vi "FSK - Sender.vi"(8 "error in (no error)":errorcluster, 11 "Queues":T1) -> (0 "error out":errorcluster)   [LabVIEW 2013]
uses:
  <vilib>/sound2/lvsound2.llb/Sound Output Task ID.ctl
  <vilib>/sound2/lvsound2.llb/Sound Data Format.ctl
  STYPS/HDR - Queues.ctl
  <vilib>/sound2/lvsound2.llb/Sampling Mode.ctl
  <vilib>/sound2/lvsound2.llb/Sound Output Write (DBL Single).vi
panel:
  out "string":string
  in  "Play Button":bool
  out "Array":u8[](array[numeric])
  in  "data length (B)":i32=100
  in  "PROPERTIES":T4={"device ID"=0, "number of samples/ch"=2500, "task ID"=0, "sound format"={"sample rate (S/s)"=44100.0, "number of channels"=1, "bits per sample"=16}, "DATA"=[]} {"task ID" format="%.0x"}
  out "i":i32
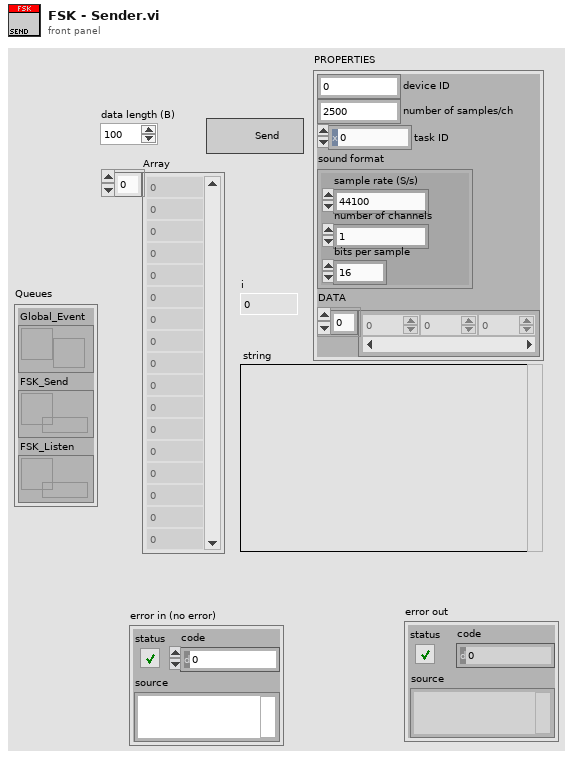
[diagram p1: front panel]
types:
  T1 = typedef "HDR - Queues.ctl" = cluster{"Global_Event":refnum<user-event>, "FSK_Send":refnum<queue>, "FSK_Listen":refnum<queue>}
  T2 = typedef "Sound Output Task ID.ctl" = u32
  T3 = typedef "Sound Data Format.ctl" = cluster{"sample rate (S/s)":dbl, "number of channels":i32, "bits per sample":i32}
  T4 = cluster{"device ID":u32, "number of samples/ch":i32, "task ID":T2, "sound format":T3, "DATA":dbl[]}
  T5 = typedef "Sampling Mode.ctl" = i32
  T6 = typedef "FSK_OBJ - PROP.ctl" = cluster{"rate (bit/s)":dbl, "bp (Bit Period)":dbl, "f1%":dbl, "f2%":dbl, "f1 (1 Freq)":dbl, "f2 (0 Freq)":dbl, "t (Time arry)":dbl[], "y1 (f1 cos arry)":dbl[], "y2 (f2 cos arry)":dbl[], "data length (B)":i32, "data size":i32, "sample size":dbl}
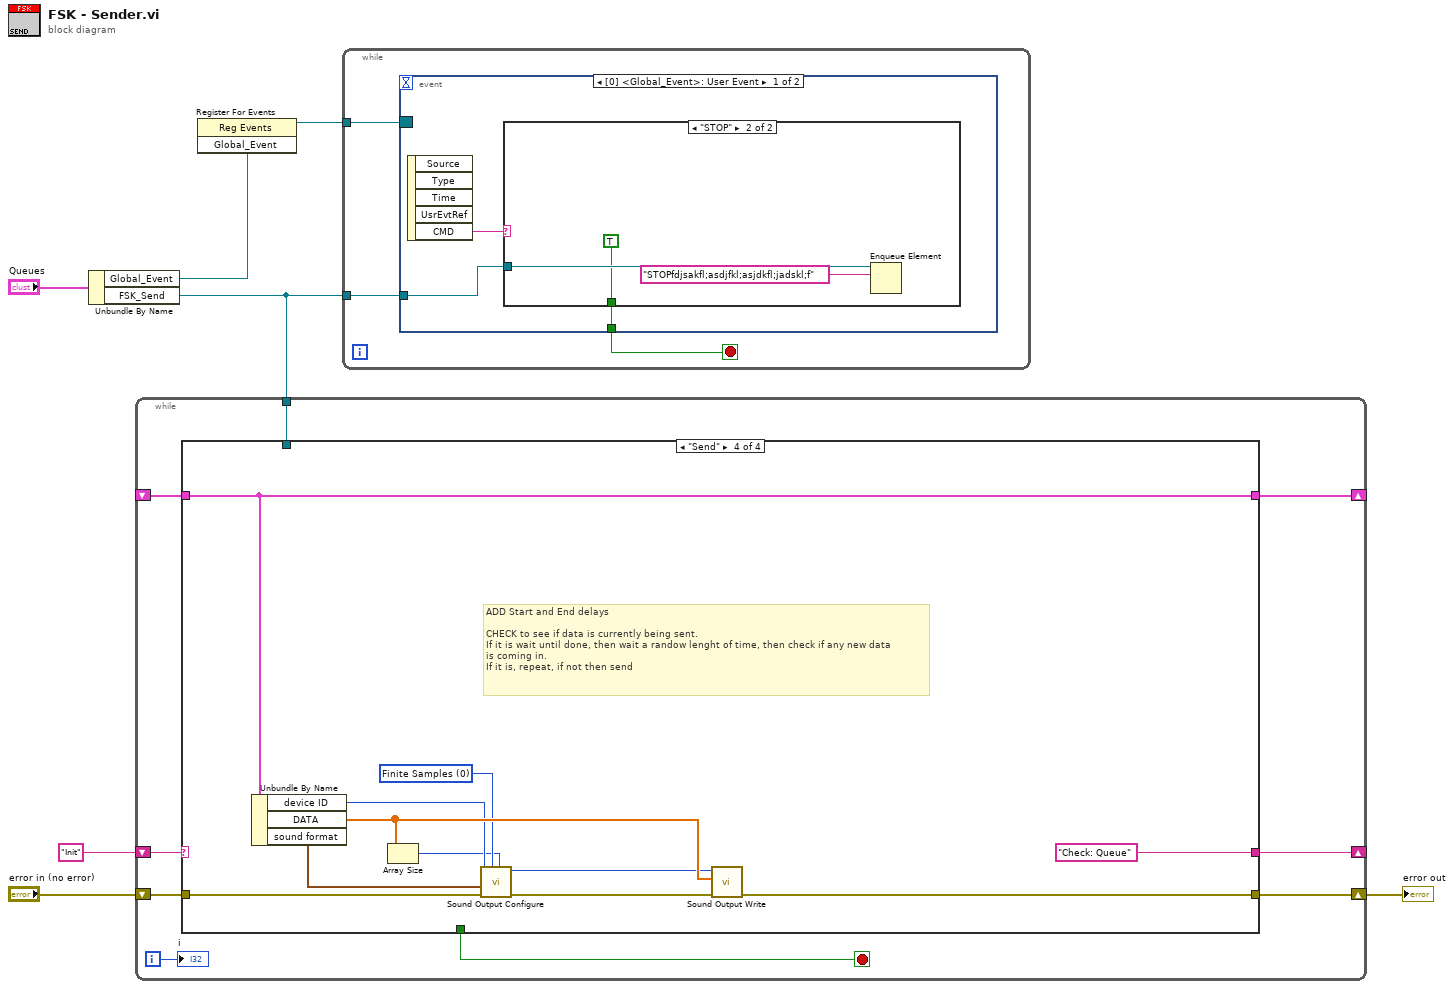
[diagram p0: block diagram]
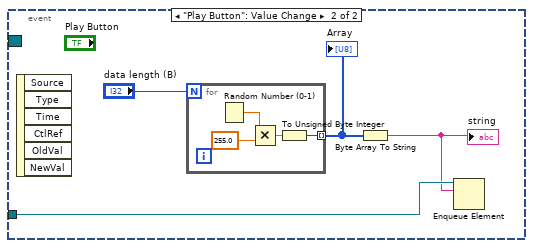
[diagram p3: hidden frame]
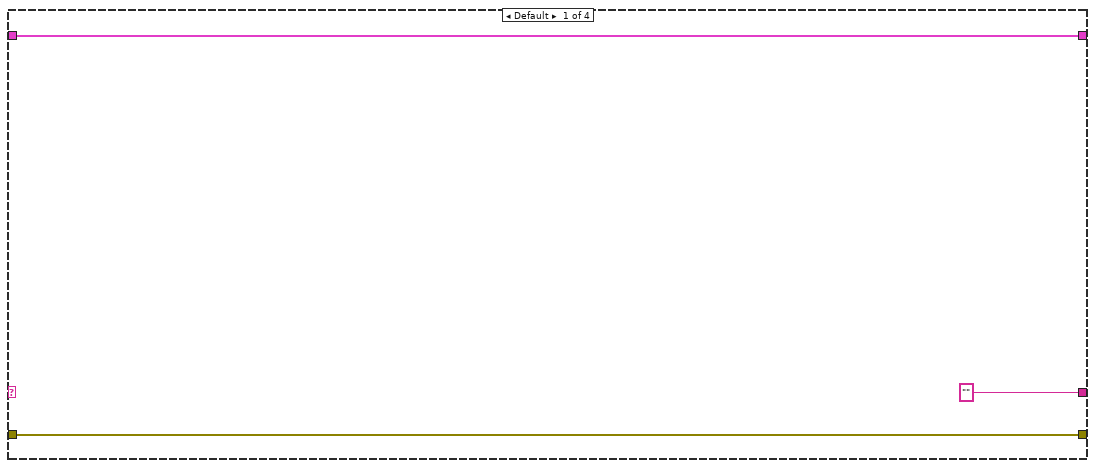
[diagram p4: hidden frame]
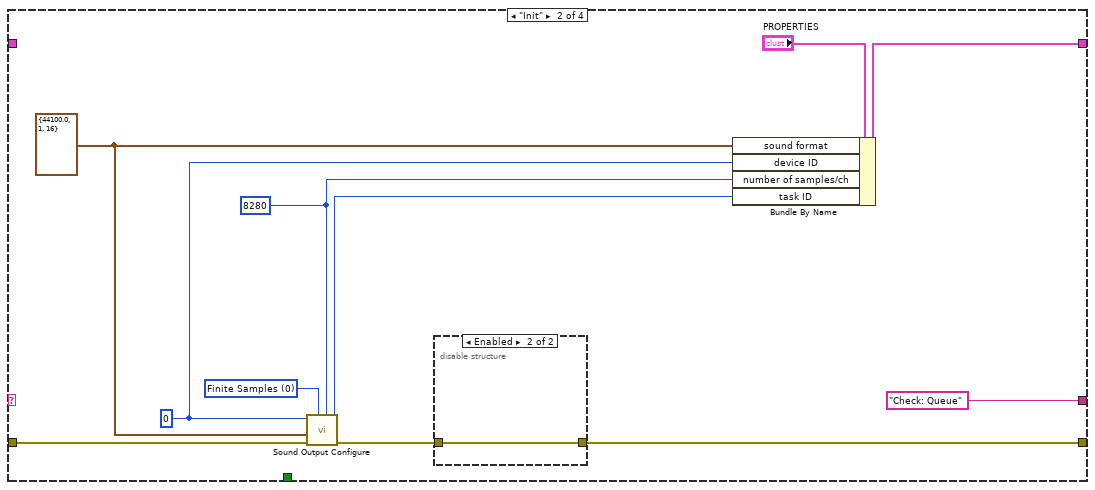
[diagram p5: hidden frame]
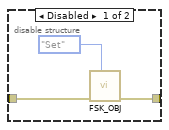
[diagram p6: hidden frame]
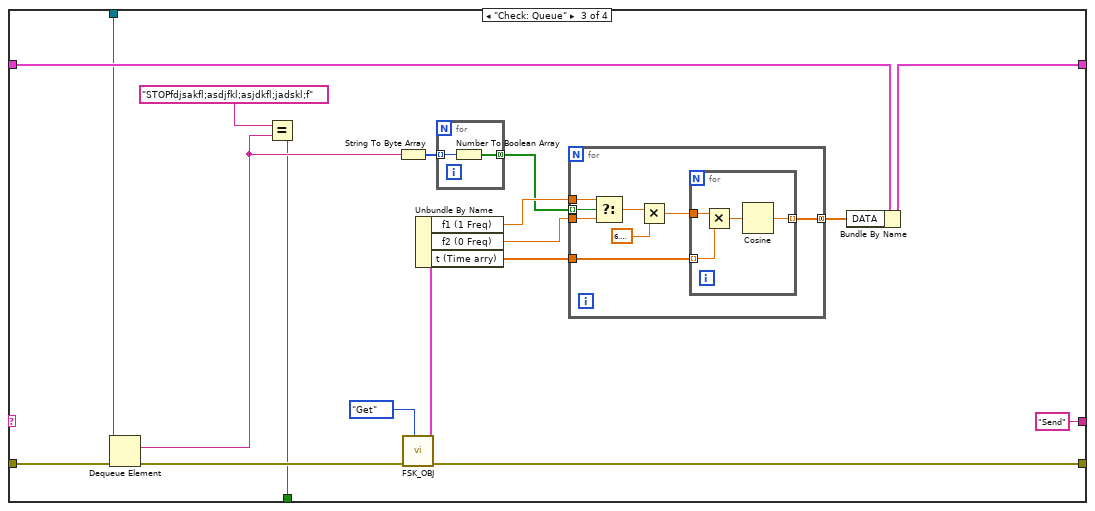
[diagram p7: hidden frame]
diagram:
  n1 = Unbundle By Name("Queues") -> ("Global_Event"=w3:refnum<user-event>, "FSK_Send"=w5:refnum<queue>)
  n2 = while {
    shift-right: [w13] -> _
    shift-left: "Init" -> [w14]
    shift-right: [w12] -> w1
    shift-left: "error in (no error)" -> [w16]
    shift-right: [w11] -> _
    shift-left: _ -> [w10]
    tunnel: w5 -> [w9]
    i -> [w15]
    stop <- w8 stop-if-true
    n3 = case shown="\"Send\"" w14 {
      tunnel: w16 -> [w19 w29 w42 w73]
      tunnel: ["" "Check: Queue" "Send" "Check: Queue"] -> w13
      tunnel: [w19 w20 w50 w76] -> w12
      tunnel: [w18 w26 w40 w75] -> w11
      tunnel: w10 -> [w18 _ w52 w75]
      tunnel: w9 -> [_ _ w38 _]
      tunnel: [_ _ w35 _] -> w8
      frame Default {
      }
      frame "Init" {
        w23 = u32 0 ("device ID")
        w24 = T3 {"sample rate (S/s)"=44100.0, "number of channels"=1, "bits per sample"=16} ("sound format")
        w25 = 8280 ("number of samples/ch")
        w30 = T5 0 items=["Finite Samples", "Continuous Samples"] ("sample mode")
        n4 = call <vilib>:"Sound Output Configure.vi"("number of samples/ch"=w25, "sample mode"=w30, "error in (no error)"=w29, "sound format"=w24, "device ID"=w23) -> ("error out"=w21:errorcluster, "task ID"=w22:T2)  [unwired: 5 in]
        n5 = disable-structure shown="Enabled" {
          disable-tunnel: w21 -> [w33 w34]
          disable-tunnel: [w32 w34] -> w20
          frame Disabled {
            n6 = call "FSK_OBJ.vi"("Mode"=enum16{"Get", "Set"}."Set", "error in"=w33) -> ("error out"=w32:errorcluster)  [unwired: 8 in, 1 out]
          }
          frame Enabled {
          }
        }
        n7 = Bundle By Name(cluster="PROPERTIES", "sound format"=w24, "device ID"=w23, "number of samples/ch"=w25, "task ID"=w22) -> (w26:T4)
      }
      frame "Check: Queue" {
        n8 = Dequeue Element(queue=w38, error in (no error)=w42) -> (element=w37:string, error out=w41:errorcluster)  [unwired: 1 in, 2 out]
        n9 = Equal?(x="STOPfdjsakfl;asdjfkl;asjdkfl;jadskl;f" ("element"), y=w37) -> (x = y?=w35:bool)
        n10 = String To Byte Array(string=w37) -> (unsigned byte array=w44:u8[])
        n11 = call "FSK_OBJ.vi"("Mode"=enum16{"Get", "Set"}."Get", "error in"=w41) -> ("error out"=w50:errorcluster, "PROPERTIES OUT"=w48:T6)  [unwired: 8 in]
        n12 = Unbundle By Name(w48) -> ("f1 (1 Freq)"=w46:dbl, "f2 (0 Freq)"=w45:dbl, "t (Time arry)"=w47:dbl[])
        n13 = for {
          tunnel: w44 -> [w54] mode=indexing
          tunnel: [w53] -> w43 mode=concatenating
          n14 = Number To Boolean Array(number=w54) -> (Boolean array=w53:bool[])
        }
        n15 = for {
          tunnel: w43 -> [w62] mode=indexing
          tunnel: w47 -> [w56]
          tunnel: w46 -> [w61]
          tunnel: w45 -> [w60]
          tunnel: [w55] -> w39 mode=concatenating
          n16 = Select(t=w61, s=w62, f=w60) -> (s? t:f=w59:dbl)
          n17 = Multiply(x=w59, y=6.283185307179586) -> (x*y=w57:dbl)
          n18 = for {
            tunnel: w57 -> [w66]
            tunnel: w56 -> [w65] mode=indexing
            tunnel: [w63] -> w55 mode=indexing
            n19 = Multiply(x=w66, y=w65) -> (x*y=w64:dbl)
            n20 = Cosine(x=w64) -> (cos(x)=w63:dbl)
          }
        }
        n21 = Bundle By Name(cluster=w52, "DATA"=w39) -> (w40:T4)
      }
      frame "Send" {
        w69 = T5 0 items=["Finite Samples", "Continuous Samples"] ("sample mode")
        # "ADD Start and End delays\n\nCHECK to see if data is currently being sent.\nIf it is wait until done, then wait a randow lenght of time, then check if any new data\nis coming in.\nIf it is, repeat, if not then send"
        n22 = Unbundle By Name(w75) -> ("device ID"=w70:u32, "DATA"=w74:dbl[], "sound format"=w67:T3)
        n23 = Array Size(array=w74) -> (size(s)=w68:i32)
        n24 = call <vilib>:"Sound Output Configure.vi"("number of samples/ch"=w68, "sample mode"=w69, "error in (no error)"=w73, "sound format"=w67, "device ID"=w70) -> ("error out"=w72:errorcluster, "task ID"=w71:T2)  [unwired: 5 in]
        n25 = call-poly <vilib>:"Sound Output Write.vi"("error in (no error)"=w72, "data"=w74, "task ID"=w71) -> ("error out"=w76:errorcluster)  [unwired: 7 in, 1 out]
      }
    }
    "i" <- w15
  }
  "error out" <- w1
  n26 = register-events(w3) -> (reference out=w2:refnum<event-registration>)  [unwired: 2 in, 1 out]
  n27 = while {
    tunnel: w5 -> [w80]
    tunnel: w2 -> [w79]
    stop <- w78 stop-if-true
    n28 = event shown="[0] <Global_Event>: User Event" {
      selector: w79 -> [_ _]
      dyn-events: _ -> [_ _]
      timeout: _ -> [_ _]
      tunnel: w80 -> [w81 w89]
      tunnel: [w82 _] -> w78
      event User Event {
        n29 = event-data() -> ("CMD"=w83:string)  [unwired: 1 in, 4 out]
        n30 = case shown="\"STOP\"" w83 {
          tunnel: [_ TRUE] -> w82
          tunnel: w81 -> [_ w86]
          frame Default {
          }
          frame "STOP" {
            n31 = Enqueue Element(queue=w86, element="STOPfdjsakfl;asdjfkl;asjdkfl;jadskl;f") -> ()  [unwired: 2 in, 3 out]
          }
        }
      }
      event "Play Button": Value Change {
        n32 = event-data() -> ()  [unwired: 1 in, 6 out]
        n33 = for {
          N: "data length (B)" -> [_]
          tunnel: [w91] -> w88 mode=indexing
          n34 = Random Number (0-1)() -> (number: 0 to 1=w94:dbl)
          n35 = Multiply(x=w94, y=255.0) -> (x*y=w92:dbl)
          n36 = To Unsigned Byte Integer(number=w92) -> (unsigned 8bit integer=w91:u8)
        }
        "Array" <- w88
        n37 = Byte Array To String(unsigned byte array=w88) -> (string=w87:string)
        "string" <- w87
        n38 = Enqueue Element(queue=w89, element=w87) -> ()  [unwired: 2 in, 3 out]
      }
    }
  }
